vi "ClientIndividualUDP.vi"(0 "UDP Connection ID":refnum<k16>, 1 "Rover Inputs":cluster{"Left PWM":i32, "Right PWM":i32}={"Left PWM"=1500, "Right PWM"=1500}, 2 "Remote Port #":i32=61540, 3 "error in (no error)":errorcluster, 4 "Robot Symbol":string) -> (5 "connection ID out":refnum<k16>, 6 "Robot Heading":i32, 7 "error out":errorcluster)   [LabVIEW 2012]
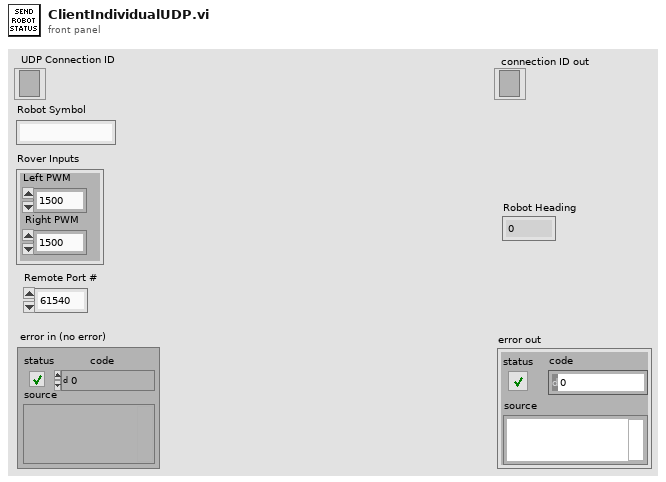
[diagram p1: front panel]
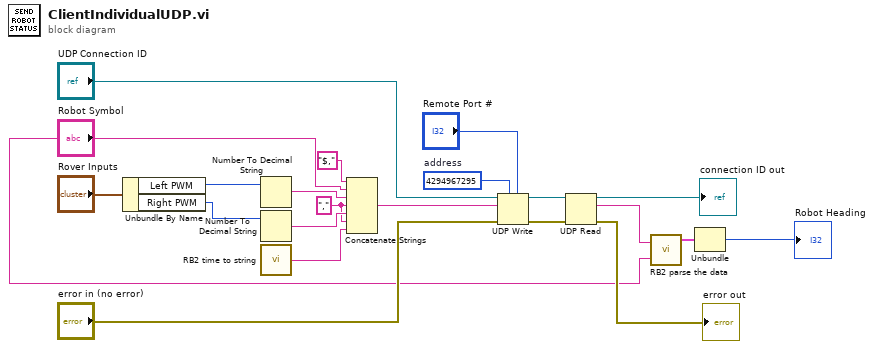
[diagram p0: block diagram]
diagram:
  w12 = u32 4294967295  # address
  w17 = "," ("string")
  n1 = Unbundle By Name("Rover Inputs") -> ("Left PWM"=w20:i32, "Right PWM"=w19:i32)
  n2 = Number To Decimal String(number=w20) -> (decimal integer string=w16:string)  [unwired: 1 in]
  n3 = Number To Decimal String(number=w19) -> (decimal integer string=w18:string)  [unwired: 1 in]
  n4 = call "RB2 time to string.vi"() -> ("time string"=w15:string)  [unwired: 1 in]
  n5 = Concatenate Strings("$," ("string"), "Robot Symbol", w16, w17, w18, w17, w15) -> (w13:string)
  n6 = UDP Write(address=w12, port or service name="Remote Port #", connection ID="UDP Connection ID", data in=w13, 8:"error in (no error)") -> (error out=w7:errorcluster, 3:w8:refnum<k16>)  [unwired: 1 in]
  n7 = UDP Read(connection ID=w8, 8:w7) -> (data out=w3:string, error out=→"error out":errorcluster, 3:→"connection ID out":refnum<k16>)  [unwired: 2 in, 2 out]
  n8 = call "RB2 parse the data.vi"("Nav String"=w3, "Jeep"="Robot Symbol") -> ("Jeep Data"=w2:cluster{"Header":string, i32, i32})  [unwired: 2 out]
  n9 = Unbundle(w2) -> (→"Robot Heading":i32)  [unwired: 2 out]
